vi "On Target.vi"(0 "Target X":i16, 1 "X Tolerance":i16, 2 "X":i16, 3 "Y":i16, 4 "Y Tolerance":i16, 5 "Target Y":i16) -> (6 "Horizontal In Range":bool, 7 "Turn Speed":dbl, 8 "Arm Lift Speed":dbl)   [LabVIEW 2015]
panel:
  out "Vertical In Range":bool
  in  "Turn Speed in":dbl=0.4
  in  "Arm Lift Speed in":dbl=0.4
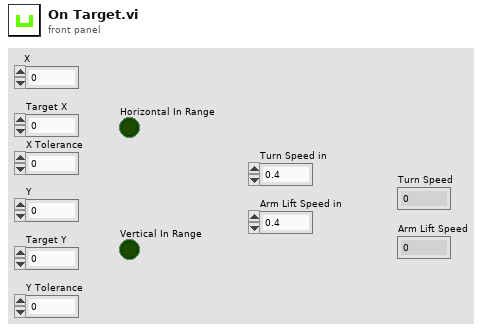
[diagram p1: front panel]
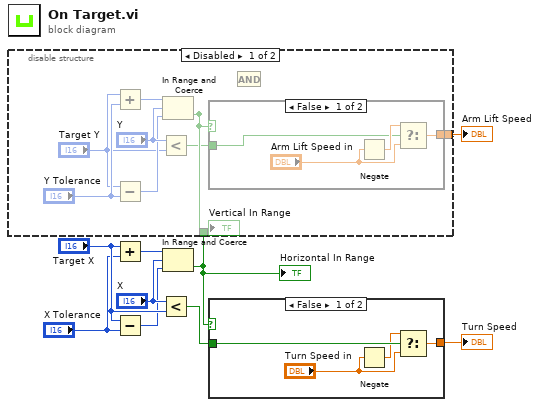
[diagram p0: block diagram]
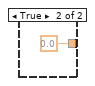
[diagram p2: hidden frame]
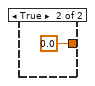
[diagram p4: hidden frame]
diagram:
  n1 = Add(x="Target X", y="X Tolerance") -> (x+y=w5:i16)
  n2 = Subtract(x="Target X", y="X Tolerance") -> (x-y=w3:i16)
  n3 = Less?(x="X", y="Target X") -> (x < y?=w8:bool)
  n4 = In Range and Coerce(upper limit=w5, x="X", lower limit=w3) -> (In Range?=w1:bool)  [unwired: 1 out]
  "Horizontal In Range" <- w1
  n5 = disable-structure shown="Disabled" {
    disable-tunnel: [w16 _] -> w6
    disable-tunnel: w1 -> [w10 _]
    frame Disabled {
      n6 = Add(x="Target Y", y="Y Tolerance") -> (x+y=w13:i16)
      n7 = Subtract(x="Target Y", y="Y Tolerance") -> (x-y=w12:i16)
      n8 = Less?(x="Y", y="Target Y") -> (x < y?=w17:bool)
      n9 = In Range and Coerce(upper limit=w13, x="Y", lower limit=w12) -> (In Range?=w18:bool)  [unwired: 1 out]
      "Vertical In Range" <- w18
      n10 = case shown="False" w18 {
        tunnel: [w21 0.0] -> w16
        tunnel: w17 -> [w20 _]
        frame False {
          n11 = Negate(x="Arm Lift Speed in") -> (-x=w22:dbl)
          n12 = Select(t=w22, s=w20, f="Arm Lift Speed in") -> (s? t:f=w21:dbl)
        }
        frame True {
        }
      }
      n13 = And() -> ()  [unwired: 2 in, 1 out]
    }
    frame Enabled {
    }
  }
  "Arm Lift Speed" <- w6
  n14 = case shown="False" w1 {
    tunnel: [w27 0.0] -> w7
    tunnel: w8 -> [w26 _]
    frame False {
      n15 = Negate(x="Turn Speed in") -> (-x=w24:dbl)
      n16 = Select(t=w24, s=w26, f="Turn Speed in") -> (s? t:f=w27:dbl)
    }
    frame True {
    }
  }
  "Turn Speed" <- w7
